vi "显示测试结果-放料点坐标.vi"(9 "当前放料点":T1, 11 "Img输入":T2) -> ()   [LabVIEW 2014]
uses:
  <vilib>/vision/Image Controls.llb/IMAQ Image.ctl
  Controls/XYZRPos.ctl
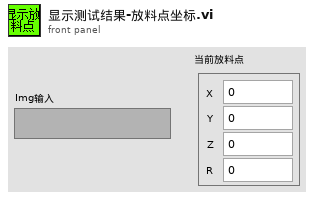
[diagram p1: front panel]
types:
  T1 = typedef "XYZRPos.ctl" = cluster{"X":dbl, "Y":dbl, "Z":dbl, "R":dbl}
  T2 = typedef "IMAQ Image.ctl" = refnum<image>
  T3 = cluster{"Desired Font (Application)":enum16{"User-specified Font", "Application Font", "System Font", "Dialog Font"}, "[User-specified Font]":cluster{"Font Name":string, "Size":i16, "Strikeout?":bool, "Italic?":bool, "Underline?":bool, "Outline?":bool, "Shadow?":bool, "Bold?":bool, "Rotation Angle":dbl}, "Horizontal Alignment":i16, "Vertical Alignment":i16}
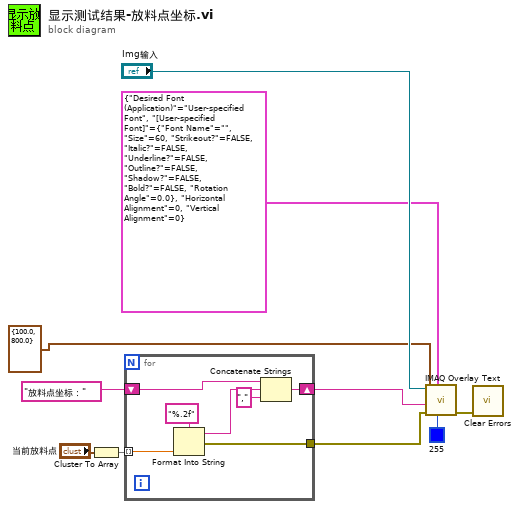
[diagram p0: block diagram]
diagram:
  n1 = Cluster To Array(cluster="当前放料点") -> (array=w1:dbl[])
  n2 = for {
    tunnel: [w15] -> w6
    shift-right: [w14] -> w4
    shift-left: "放料点坐标：" -> [w17]
    tunnel: w1 -> [w11] mode=indexing
    n3 = Format Into String(format string="%.2f" ("格式字符串"), w11) -> (resulting string=w13:string, error out=w15:errorcluster)  [unwired: 2 in]
    n4 = Concatenate Strings(w17, w13, "," ("字符串")) -> (w14:string)
  }
  n5 = call "IMAQ Overlay Text"("Text Color (black)"=u32 255, "Font, Size & Style"=T3 {"Desired Font (Application)"=enum."User-specified Font", "[User-specified Font]"={"Font Name"="", "Size"=60, "Strikeout?"=FALSE, "Italic?"=FALSE, "Underline?"=FALSE, "Outline?"=FALSE, "Shadow?"=FALSE, "Bold?"=FALSE, "Rotation Angle"=0.0}, "Horizontal Alignment"=0, "Vertical Alignment"=0}, "error in (no error)"=w6, "String"=w4, "Origin"=cluster{dbl, "Numeric":dbl} {100.0, "Numeric"=800.0}, "Image"="Img输入") -> ("error out"=w5:errorcluster)  [unwired: 4 in, 1 out]
  n6 = call <vilib>:"Clear Errors.vi"("error in (no error)"=w5) -> ()  [unwired: 5 in, 2 out]
